vi "New (Array).vi"(9 "aggregation method (all)":T3=enum."All", 10 "match behavior (keep)":T2, 11 "scope info":T1(array[cluster])) -> (3 "basic scope":refnum<class "Basic.lvclass">)   [LabVIEW 2018, in "GLog.lvlib" / "Basic.lvclass"]
uses:
  Basic.lvclass
  C:/Users/Colin/Documents/software_projects/glog/src/api/extension/filter_interface/Filter.lvclass
  extension/filter_interface/Aggregation Method.ctl
  extension/filter_interface/Match Behavior.ctl
  Basic.lvclass/Basic.ctl
  extension/filter_interface/Filter.lvclass/Filter.ctl
  extension/filter_interface/Filter.lvclass
  GLog.lvlib
panel:
  # "Connector Pane"
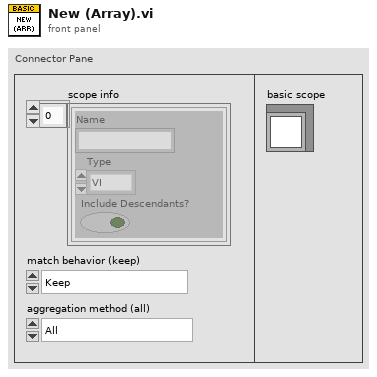
[diagram p1: front panel]
types:
  T1 = cluster{"Name":string, "Type":enum16{"VI", "Library", "Class"}, "Include Descendants?":bool}[]
  T2 = typedef "GLog.lvlib/Match Behavior.ctl" = enum16{"Keep", "Discard"}
  T3 = typedef "GLog.lvlib/Aggregation Method.ctl" = enum16{"Any", "Only", "All", "None"}
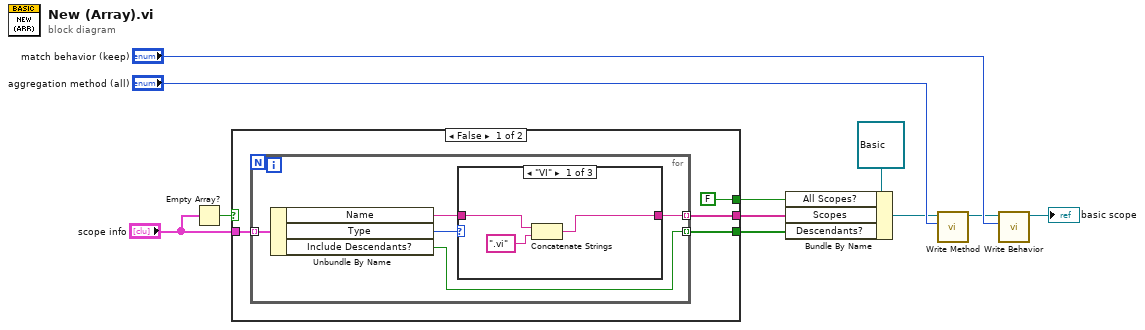
[diagram p0: block diagram]
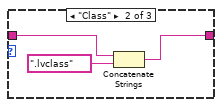
[diagram p2: hidden frame]
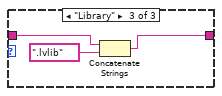
[diagram p3: hidden frame]
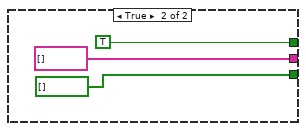
[diagram p4: hidden frame]
diagram:
  n1 = Empty Array?(array="scope info") -> (empty?=w7:bool)
  n2 = case shown="False" w7 {
    tunnel: "scope info" -> [w15 _]
    tunnel: [FALSE TRUE] -> w10
    tunnel: [w14 string[] []] -> w9
    tunnel: [w12 bool[] []] -> w8
    frame False {
      n3 = for {
        tunnel: w15 -> [w18] mode=indexing
        tunnel: [w20] -> w14 mode=indexing
        tunnel: [w17] -> w12 mode=indexing
        n4 = Unbundle By Name(w18) -> ("Name"=w16:string, "Type"=w19:enum16{"VI", "Library", "Class"}, "Include Descendants?"=w17:bool)
        n5 = case shown="\"VI\"" w19 {
          tunnel: [w22 w24 w28] -> w20
          tunnel: w16 -> [w21 w25 w27]
          frame "VI" {
            n6 = Concatenate Strings(w21, ".vi") -> (w22:string)
          }
          frame "Class" {
            n7 = Concatenate Strings(w25, ".lvclass") -> (w24:string)
          }
          frame "Library" {
            n8 = Concatenate Strings(w27, ".lvlib") -> (w28:string)
          }
        }
      }
    }
    frame True {
    }
  }
  n9 = Bundle By Name(cluster=refnum<class "Basic.lvclass"> refnum ("VI Scope out"), "All Scopes?"=w10, "Scopes"=w9, "Descendants?"=w8) -> (w4:refnum<class "Basic.lvclass">)
  n10 = call "Write Method.vi"("Method"="aggregation method (all)", "Filter in"=w4) -> ("Filter out"=w3:refnum<class "Basic.lvclass">)  [unwired: 9 in]
  n11 = call "Write Behavior.vi"("match behavior"="match behavior (keep)", "Filter in"=w3) -> ("Filter out"=→"basic scope":refnum<class "Basic.lvclass">)  [unwired: 9 in]
